vi "Reset Steps.vi"(8 "error in (no error)":errorcluster, 11 "Double Scanner in":refnum<class "Double Scanner.lvclass">) -> (0 "error out":errorcluster, 3 "Double Scanner out":refnum<class "Double Scanner.lvclass">)   [LabVIEW 2012, in "Double Scanner.lvclass"]
uses:
  Double Scanner.lvclass
  Scanner/Scanner.lvclass
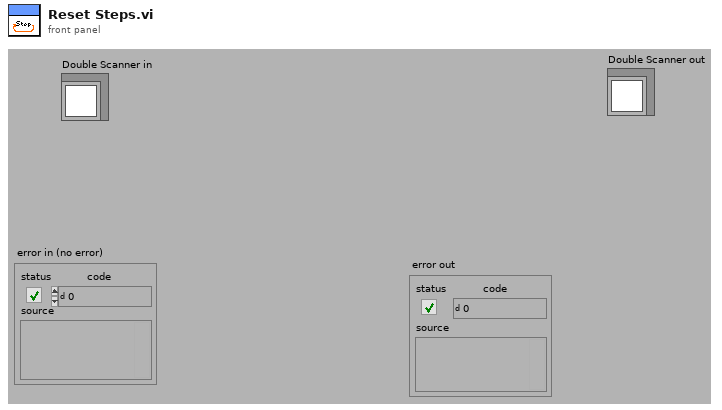
[diagram p1: front panel]
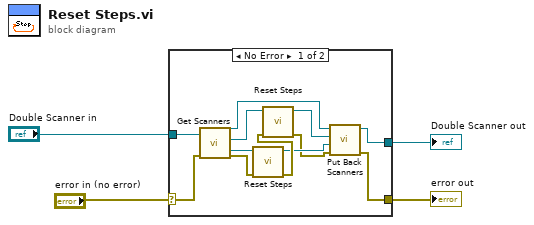
[diagram p0: block diagram]
diagram:
  n1 = case shown="No Error" "error in (no error)" {
    selector: "error in (no error)" -> [w15 w18]
    tunnel: [w5 w17] -> w4
    tunnel: "Double Scanner in" -> [w16 w17]
    tunnel: [w6 w18] -> w1
    frame No Error {
      n2 = call-dynamic "Get Scanners.vi"("error in (no error)"=w15, "Double Scanner in"=w16) -> ("error out"=w12:errorcluster, "Scanner 2 out"=w13:refnum<class "Scanner.lvclass">, "Scanner 1 out"=w14:refnum<class "Scanner.lvclass">, "Double Scanner out"=w10:refnum<class "Double Scanner.lvclass">)  [unwired: 6 in]
      n3 = call-dynamic "Reset Steps.vi"("error in (no error)"=w12, "Scanner in"=w13) -> ("error out"=w11:errorcluster, "Scanner out"=w8:refnum<class "Scanner.lvclass">)  [unwired: 8 in]
      n4 = call-dynamic "Reset Steps.vi"("error in (no error)"=w11, "Scanner in"=w14) -> ("error out"=w7:errorcluster, "Scanner out"=w9:refnum<class "Scanner.lvclass">)  [unwired: 8 in]
      n5 = call-dynamic "Put Back Scanners.vi"("error in (no error)"=w7, "Scanner 2 in"=w8, "Scanner 1 in"=w9, "Double Scanner in"=w10) -> ("error out"=w6:errorcluster, "Double Scanner out"=w5:refnum<class "Double Scanner.lvclass">)  [unwired: 6 in]
    }
    frame Error {
    }
  }
  "Double Scanner out" <- w4
  "error out" <- w1
